vi "ChunkBuffer_subvi.vi"(9 "Array in":dbl[](array[numeric]), 10 "Chunk Length":i32, 11 "New Chunk in":dbl[](array[numeric])) -> (3 "Array out":dbl[](array[numeric]))   [LabVIEW 2019]
panel:
  out "x+y":i32
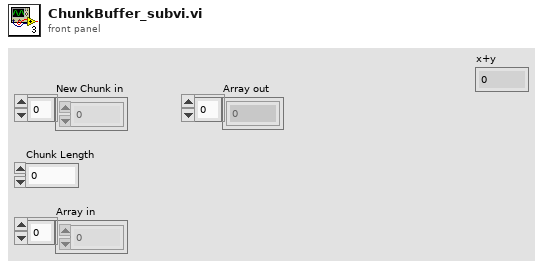
[diagram p1: front panel]
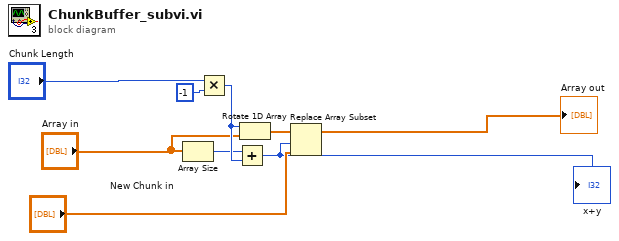
[diagram p0: block diagram]
diagram:
  n1 = Array Size(array="Array in") -> (size(s)=w1:i32)
  n2 = Multiply(x="Chunk Length", y=-1) -> (x*y=w7:i32)
  n3 = Add(x=w1, y=w7) -> (x+y=w4:i32)
  "x+y" <- w4
  n4 = Rotate 1D Array(1:"Array in", 2:w7) -> (0:w3:dbl[])
  n5 = Replace Array Subset "Replace Array Subset"(array=w3, new element="New Chunk in", index=w4) -> (→"Array out":dbl[])
